vi "Can_Add.vi"(8 "error in (no error)":errorcluster, 11 "IB_Tree_Item_Proj_Folder_Sync in":refnum<class "IB_Tree_Item_Proj_Folder_Sync.lvclass">) -> (0 "error out":errorcluster, 2 "can add?":bool, 3 "IB_Tree_Item_Proj_Folder_Sync out":refnum<class "IB_Tree_Item_Proj_Folder_Sync.lvclass">)   [LabVIEW 2020, in "IB_Tree_Item_Proj_Folder_Sync.lvclass"]
uses:
  <vilib>/AppBuilder/IB_Classes/Tree_Item_Proj_Folder_Sync/IB_Tree_Item_Proj_Folder_Sync.lvclass
  <vilib>/AppBuilder/IB_Classes/Tree_Item_Proj_Folder_Sync/IB_Tree_Item_Proj_Folder_Sync.lvclass/IB_Tree_Item_Proj_Folder_Sync.ctl
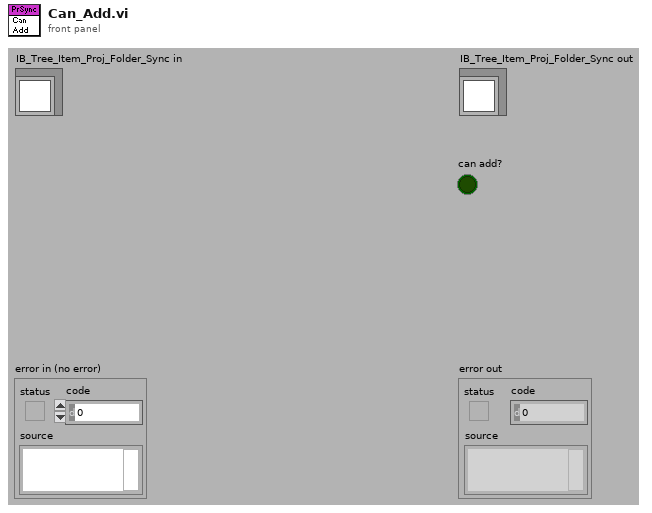
[diagram p1: front panel]
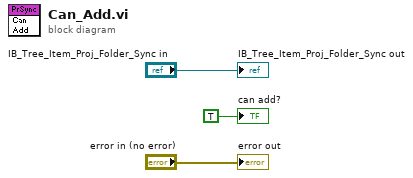
[diagram p0: block diagram]
diagram:
  "error out" <- "error in (no error)"
  "IB_Tree_Item_Proj_Folder_Sync out" <- "IB_Tree_Item_Proj_Folder_Sync in"
  "can add?" <- TRUE ("can add?")
